vi "QA_Sub.vi"(0 "U":dbl[](array[numeric]) format="%.2f", 2 "W":dbl[](array[numeric]) format="%.2f", 3 "T":dbl[](array[numeric]) format="%.2f") -> ()   [LabVIEW 2010]
uses:
  Controls/Analysis_type_Enum.ctl
  <vilib>/Utility/file.llb/Write To Spreadsheet File (DBL).vi
  <vilib>/Analysis/NI_AALBase.lvlib
panel:
  out "Loop Frame 1":i32
  out "Loop Frame 0":i32
  out "Analysis type":T1
  in  "LDA data?":bool
  in  "QA results file":path
  out "Quadrant shear totals":dbl[](array[numeric]) format="%.3f"
  out "Quadrant 'Hits' Count":dbl[](array[numeric])
  out "u'w' (bar) total":dbl format="%.3f"
  in  "H":dbl format="%.2f"
  out "XY Graph":cluster{dbl[], dbl[]}(graph)
  in  "u', w' data file":path
  # "Quadrant Analysis Subroutine for Two-Component Velocity Data"
  # "Version 1.2 -RR"
  # "Threshold,"
  # "- FOR MANUAL ENTRY -"
  # "- FOR PLUG-IN USE -"
  # "- FILES TO CREATE -"
  # "- ANALYSIS (OUTPUT) -"
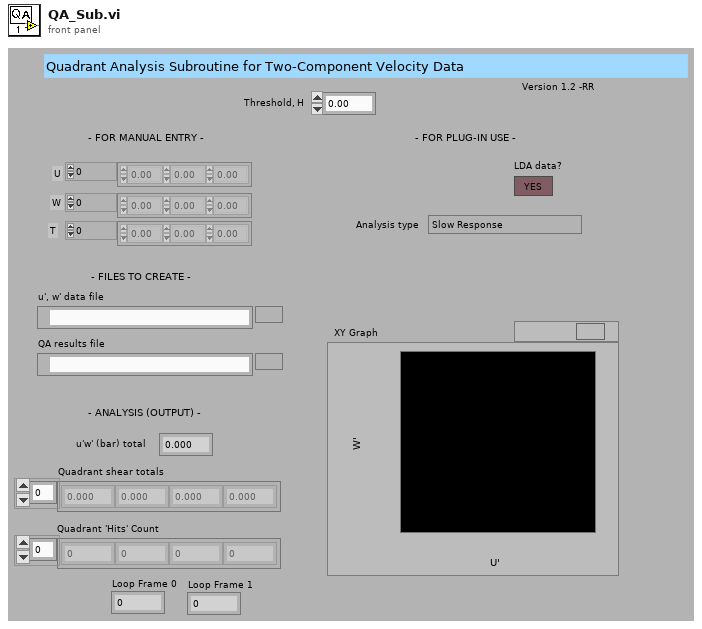
[diagram p1: front panel]
types:
  T1 = typedef "Analysis_type_Enum.ctl" = enum16{"Slow Response", "Fast Response", "Weighted Fast Response", "Fast FID", "Weighted Fast FID", "Cross Wire", "Weighted Cross Wire", "Weighted LDA"}
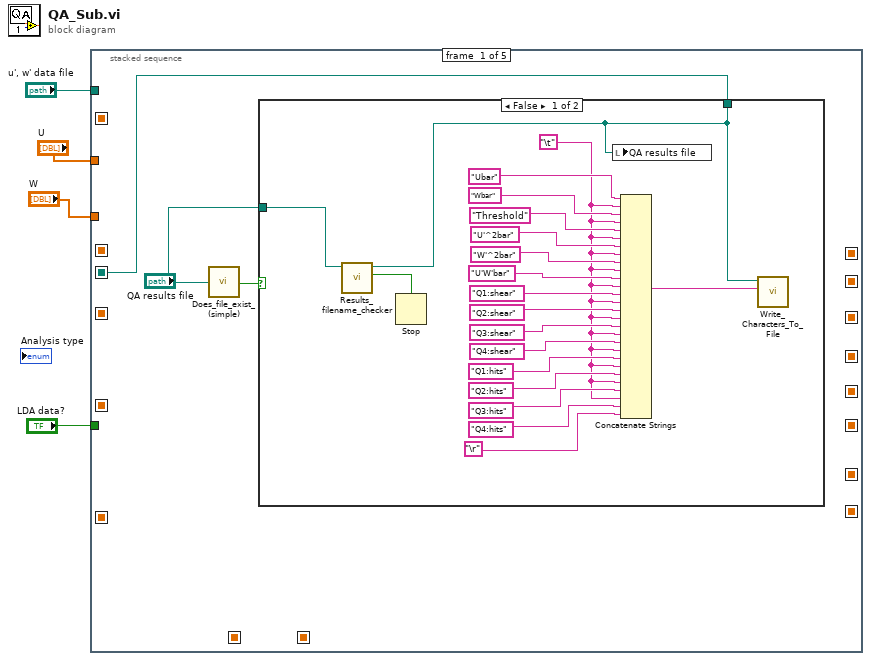
[diagram p0: block diagram]
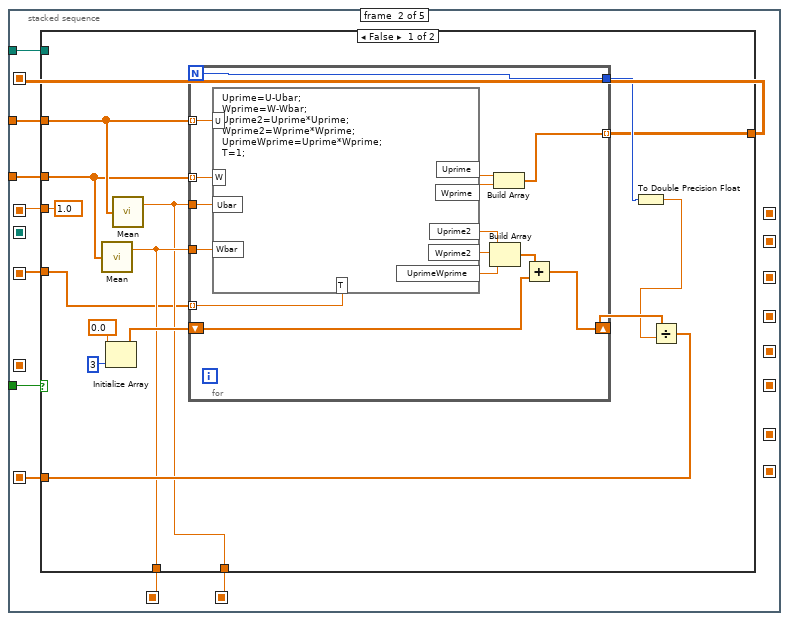
[diagram p3: hidden frame]
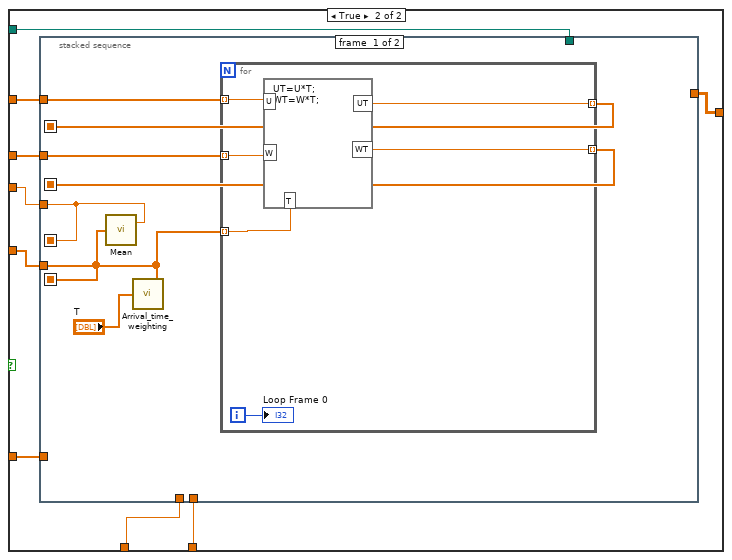
[diagram p4: hidden frame]
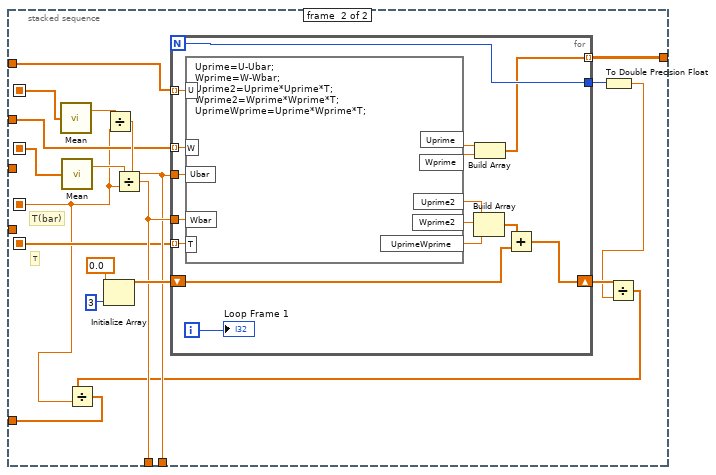
[diagram p5: hidden frame]
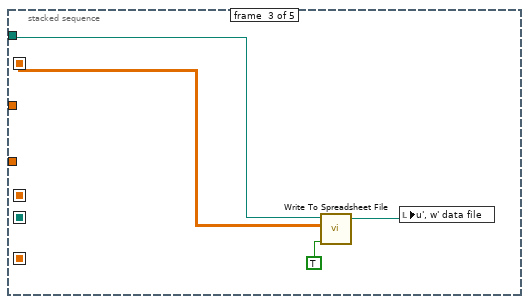
[diagram p6: hidden frame]
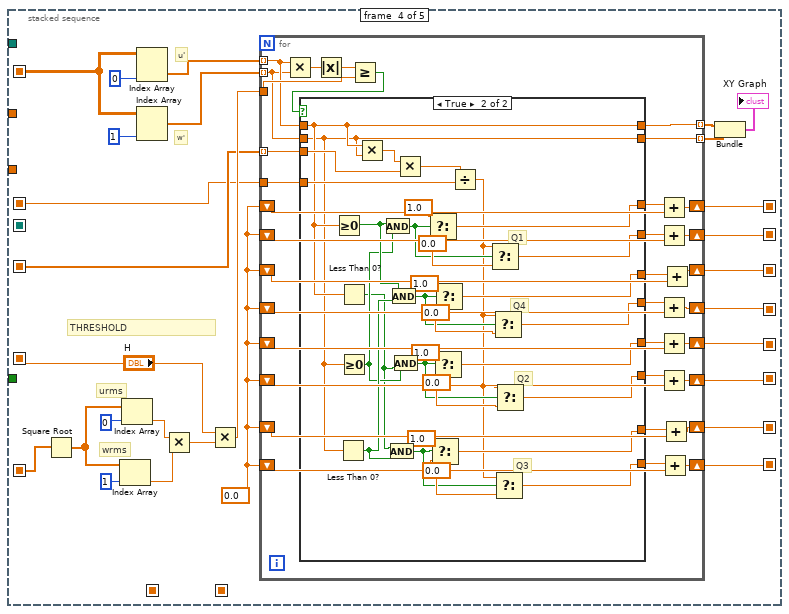
[diagram p7: hidden frame]
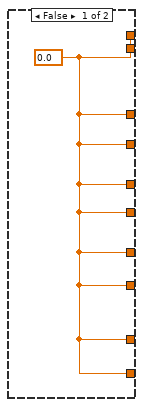
[diagram p8: hidden frame]
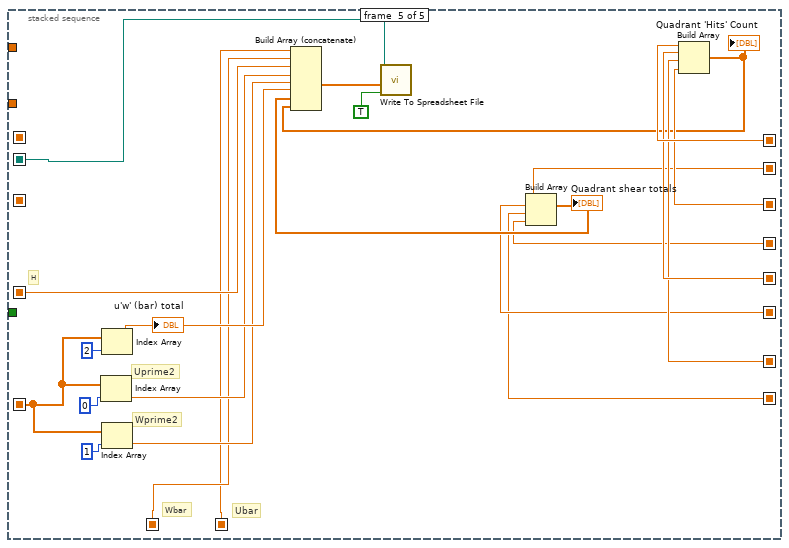
[diagram p9: hidden frame]
diagram:
  n1 = stacked-sequence {
    seq-local: [_ w37 _ _ _] -> [_ _ _ w133 w232]
    seq-local: [_ _ _ w140 _] -> [_ _ _ _ w238]
    seq-local: [_ _ _ w141 _] -> [_ _ _ _ w244]
    seq-local: [_ _ _ w139 _] -> [_ _ _ _ w241]
    seq-local: [_ _ _ w138 _] -> [_ _ _ _ w235]
    seq-local: [_ _ _ w137 _] -> [_ _ _ _ w243]
    seq-local: [_ _ _ w136 _] -> [_ _ _ _ w237]
    seq-local: [_ _ _ w135 _] -> [_ _ _ _ w242]
    seq-local: [_ _ _ w134 _] -> [_ _ _ _ w236]
    seq-local: [_ _ _ "H" _] -> [_ _ _ _ w231]
    seq-local: [_ w35 _ _ _] -> [_ _ _ _ w225]
    seq-local: [_ w34 _ _ _] -> [_ _ _ _ w224]
    seq-local: [_ w33 _ _ _] -> [_ _ _ w130 _]
    seq-local: [_ w32 _ _ _] -> [_ _ _ w131 _]
    seq-local: [_ w31 _ _ _] -> [_ _ w127 w129 _]
    seq-local: [w5 _ _ _ _] -> [_ _ _ _ w223]
    tunnel: "u', w' data file" -> [_ w38 w126 _ _]
    tunnel: "LDA data?" -> [_ w36 _ _ _]
    tunnel: "U" -> [_ w30 _ _ _]
    tunnel: "W" -> [_ w29 _ _ _]
    frame #0 {
      n2 = call "Does_file_exist_(simple).vi"("Pathname"="QA results file") -> ("exists?"=w7:bool)
      n3 = case shown="False" w7 {
        tunnel: [w9 w28] -> w5
        tunnel: "QA results file" -> [w10 w28]
        frame False {
          w12 = "\t"
          n4 = call "Results_filename_checker.vi"("Results file"=w10) -> ("cancelled"=w8:bool, "Results file output"=w9:path)  [unwired: 4 in, 2 out]
          n5 = Stop(stop? (T)=w8) -> ()
          n6 = local write "QA results file"(w9) -> ()
          n7 = Concatenate Strings("Ubar", w12, "Wbar", w12, "Threshold", w12, "U'^2bar", w12, "W'^2bar", w12, "U'W'bar", w12, "Q1:shear", w12, "Q2:shear", w12, "Q3:shear", w12, "Q4:shear", w12, "Q1:hits", w12, "Q2:hits", w12, "Q3:hits", w12, "Q4:hits", "\r") -> (w11:string)
          n8 = call "Write_Characters_To_File.vi"("file path (dialog if empty)"=w9, "character string"=w11) -> ()  [unwired: 6 in, 1 out]
        }
        frame True {
        }
      }
    }
    frame #1 {
      n9 = case shown="False" w36 {
        tunnel: w38 -> [_ w76]
        tunnel: [w48 w71] -> w37
        tunnel: w30 -> [w45 w75]
        tunnel: w29 -> [w44 w74]
        tunnel: [w43 w73] -> w35
        tunnel: [w42 w72] -> w34
        tunnel: [1.0 w70] -> w33
        tunnel: [w40 w69] -> w32
        tunnel: [w39 w68] -> w31
        frame False {
          n10 = call <vilib>:"Mean.vi"("X"=w44) -> ("mean"=w43:dbl)  [unwired: 1 out]
          n11 = Initialize Array(0.0, 3) -> (w51:dbl[])
          n12 = call <vilib>:"Mean.vi"("X"=w45) -> ("mean"=w42:dbl)  [unwired: 1 out]
          n13 = for {
            N -> [w58]
            tunnel: w45 -> [w67] mode=indexing
            tunnel: w44 -> [w66] mode=indexing
            shift-right: [w59] -> w49
            shift-left: w51 -> [w60]
            tunnel: [w58] -> w47
            tunnel: w42 -> [w56]
            tunnel: w43 -> [w55]
            tunnel: [w54] -> w40 mode=indexing
            tunnel: [w53] -> w39 mode=indexing
            n14 = formula code="Uprime=U-Ubar;\nWprime=W-Wbar;\nUprime2=Uprime*Uprime;\nWprime2=Wprime*Wprime;\nUprimeWprime=Uprime*Wprime;\nT=1;"("W"=w66, "U"=w67, "Ubar"=w56, "Wbar"=w55) -> ("Uprime"=w65:dbl, "Wprime"=w64:dbl, "Uprime2"=w63:dbl, "Wprime2"=w62:dbl, "UprimeWprime"=w57:dbl, "T"=w54:dbl)
            n15 = Build Array(w63, w62, w57) -> (w61:dbl[])
            n16 = Build Array(w65, w64) -> (w53:dbl[])
            n17 = Add(x=w61, y=w60) -> (x+y=w59:dbl[])
          }
          n18 = To Double Precision Float(number=w47) -> (double precision float=w46:dbl)
          n19 = Divide(x=w49, y=w46) -> (x/y=w48:dbl[])
        }
        frame True {
          n20 = stacked-sequence {
            seq-local: [w81 _] -> [_ w104]
            seq-local: [w80 _] -> [_ w105]
            seq-local: [w79 _] -> [_ w93]
            seq-local: [w78 _] -> [_ w97]
            tunnel: w76 -> [_ _]
            tunnel: w75 -> [w83 w99]
            tunnel: w74 -> [w82 w98]
            tunnel: [_ w103] -> w73
            tunnel: [_ w100] -> w72
            tunnel: [_ w92] -> w71
            tunnel: [w79 _] -> w70
            tunnel: [w78 _] -> w69
            tunnel: [_ w90] -> w68
            frame #0 {
              n21 = call "Arrival_time_weighting.vi"("Arrival times"="T") -> ("Weighting"=w78:dbl[])
              n22 = call <vilib>:"Mean.vi"("X"=w78) -> ("mean"=w79:dbl)  [unwired: 1 out]
              n23 = for {
                tunnel: w83 -> [w89] mode=indexing
                tunnel: w82 -> [w88] mode=indexing
                tunnel: w78 -> [w87] mode=indexing
                tunnel: [w86] -> w81 mode=indexing
                tunnel: [w85] -> w80 mode=indexing
                i -> [w84]
                n24 = formula code="UT=U*T;\nWT=W*T;"("T"=w87, "U"=w89, "W"=w88) -> ("UT"=w86:dbl, "WT"=w85:dbl)
                "Loop Frame 0" <- w84
              }
            }
            frame #1 {
              # "T"
              # "T(bar)"
              n25 = call <vilib>:"Mean.vi"("X"=w104) -> ("mean"=w102:dbl)  [unwired: 1 out]
              n26 = call <vilib>:"Mean.vi"("X"=w105) -> ("mean"=w101:dbl)  [unwired: 1 out]
              n27 = Initialize Array(0.0, 3) -> (w106:dbl[])
              n28 = Divide(x=w102, y=w93) -> (x/y=w100:dbl)
              n29 = Divide(x=w101, y=w93) -> (x/y=w103:dbl)
              n30 = for {
                N -> [w115]
                tunnel: w99 -> [w124] mode=indexing
                tunnel: w98 -> [w123] mode=indexing
                shift-right: [w116] -> w95
                shift-left: w106 -> [w117]
                tunnel: [w115] -> w96
                tunnel: w100 -> [w113]
                tunnel: w103 -> [w112]
                tunnel: w97 -> [w111] mode=indexing
                tunnel: [w110] -> w90 mode=indexing
                i -> [w109]
                n31 = formula code="Uprime=U-Ubar;\nWprime=W-Wbar;\nUprime2=Uprime*Uprime*T;\nWprime2=Wprime*Wprime*T;\nUprimeWprime=Uprime*Wprime*T;"("W"=w123, "U"=w124, "Ubar"=w113, "Wbar"=w112, "T"=w111) -> ("Uprime"=w122:dbl, "Wprime"=w121:dbl, "Uprime2"=w120:dbl, "Wprime2"=w119:dbl, "UprimeWprime"=w114:dbl)
                n32 = Build Array(w120, w119, w114) -> (w118:dbl[])
                n33 = Build Array(w122, w121) -> (w110:dbl[])
                n34 = Add(x=w118, y=w117) -> (x+y=w116:dbl[])
                "Loop Frame 1" <- w109
              }
              n35 = To Double Precision Float(number=w96) -> (double precision float=w94:dbl)
              n36 = Divide(x=w95, y=w94) -> (x/y=w91:dbl[])
              n37 = Divide(x=w91, y=w93) -> (x/y=w92:dbl[])
            }
          }
        }
      }
    }
    frame #2 {
      n38 = call-poly <vilib>:"Write To Spreadsheet File.vi"("append to file? (new file:F)"=TRUE, "2D data"=w127, "file path (dialog if empty)"=w126) -> ("new file path (Not A Path if cancelled)"=w125:path)  [unwired: 5 in]
      n39 = local write "u', w' data file"(w125) -> ()
    }
    frame #3 {
      w132 = 0.0
      # "THRESHOLD"
      # "wrms"
      # "urms"
      # "w'"
      # "u'"
      n40 = Square Root(x=w133) -> (sqrt(x)=w154:dbl[])
      n41 = Index Array(array=w154, index=1) -> (element=w150:dbl)
      n42 = Index Array(array=w154, index=0) -> (element=w151:dbl)
      n43 = Index Array(array=w129, index (col)=0) -> (element=w147:dbl[])  [unwired: 1 in]
      n44 = Index Array(array=w129, index (col)=1) -> (element=w146:dbl[])  [unwired: 1 in]
      n45 = Multiply(x=w151, y=w150) -> (x*y=w148:dbl)
      n46 = Multiply(x="H", y=w148) -> (x*y=w145:dbl)
      n47 = for {
        tunnel: w147 -> [w186] mode=indexing
        tunnel: w146 -> [w185] mode=indexing
        tunnel: w145 -> [w188]
        tunnel: [w184] -> w144 mode=indexing
        tunnel: [w183] -> w143 mode=indexing
        shift-right: [w175] -> w140
        shift-left: w132 -> [w165]
        shift-right: [w182] -> w138
        shift-left: w132 -> [w163]
        shift-right: [w181] -> w136
        shift-left: w132 -> [w161]
        shift-right: [w180] -> w134
        shift-left: w132 -> [w159]
        shift-right: [w167] -> w141
        shift-left: w132 -> [w166]
        shift-right: [w174] -> w139
        shift-left: w132 -> [w164]
        shift-right: [w173] -> w137
        shift-left: w132 -> [w162]
        shift-right: [w168] -> w135
        shift-left: w132 -> [w160]
        tunnel: w131 -> [w158] mode=indexing
        tunnel: w130 -> [w157]
        n48 = Multiply(x=w186, y=w185) -> (x*y=w190:dbl)
        n49 = Absolute Value(x=w190) -> (abs(x)=w189:dbl)
        n50 = Greater Or Equal?(x=w189, y=w188) -> (x >= y?=w187:bool)
        n51 = case shown="True" w187 {
          tunnel: w186 -> [_ w195]
          tunnel: w185 -> [_ w194]
          tunnel: [w191 w195] -> w184
          tunnel: [w191 w194] -> w183
          tunnel: [w191 w206] -> w179
          tunnel: [w191 w205] -> w178
          tunnel: [w191 w204] -> w177
          tunnel: [w191 w203] -> w176
          tunnel: [w191 w202] -> w172
          tunnel: [w191 w201] -> w171
          tunnel: [w191 w200] -> w170
          tunnel: [w191 w199] -> w169
          tunnel: w158 -> [_ w196]
          tunnel: w157 -> [_ w198]
          frame False {
            w191 = 0.0
          }
          frame True {
            w219 = 0.0
            w220 = 0.0
            w221 = 0.0
            w222 = 0.0
            # "Q3"
            # "Q2"
            # "Q4"
            # "Q1"
            n52 = Greater Or Equal To 0?(x=w195) -> (x >= 0?=w214:bool)
            n53 = Less Than 0?(x=w194) -> (x < 0?=w213:bool)
            n54 = Less Than 0?(x=w195) -> (x < 0?=w211:bool)
            n55 = Greater Or Equal To 0?(x=w194) -> (x >= 0?=w212:bool)
            n56 = Multiply(x=w195, y=w194) -> (x*y=w193:dbl)
            n57 = And(x=w214, y=w212) -> (x .and. y?=w210:bool)
            n58 = And(x=w211, y=w213) -> (x .and. y?=w207:bool)
            n59 = And(x=w214, y=w213) -> (x .and. y?=w209:bool)
            n60 = And(x=w212, y=w211) -> (x .and. y?=w208:bool)
            n61 = Multiply(x=w193, y=w196) -> (x*y=w192:dbl)
            n62 = Select(t=1.0, s=w210, f=w222) -> (s? t:f=w202:dbl)
            n63 = Select(t=1.0, s=w207, f=w219) -> (s? t:f=w199:dbl)
            n64 = Select(t=1.0, s=w208, f=w220) -> (s? t:f=w200:dbl)
            n65 = Select(t=1.0, s=w209, f=w221) -> (s? t:f=w201:dbl)
            n66 = Divide(x=w192, y=w198) -> (x/y=w197:dbl)
            n67 = Select(t=w197, s=w210, f=w222) -> (s? t:f=w206:dbl)
            n68 = Select(t=w197, s=w209, f=w221) -> (s? t:f=w205:dbl)
            n69 = Select(t=w197, s=w207, f=w219) -> (s? t:f=w203:dbl)
            n70 = Select(t=w197, s=w208, f=w220) -> (s? t:f=w204:dbl)
          }
        }
        n71 = Add(x=w172, y=w166) -> (x+y=w167:dbl)
        n72 = Add(x=w179, y=w165) -> (x+y=w175:dbl)
        n73 = Add(x=w178, y=w163) -> (x+y=w182:dbl)
        n74 = Add(x=w170, y=w162) -> (x+y=w173:dbl)
        n75 = Add(x=w177, y=w161) -> (x+y=w181:dbl)
        n76 = Add(x=w176, y=w159) -> (x+y=w180:dbl)
        n77 = Add(x=w169, y=w160) -> (x+y=w168:dbl)
        n78 = Add(x=w171, y=w164) -> (x+y=w174:dbl)
      }
      n79 = Bundle(w144, w143) -> (→"XY Graph":cluster{dbl[], dbl[]})  [unwired: 1 in]
    }
    frame #4 {
      # "Wprime2"
      # "Uprime2"
      # "H"
      # "Wbar"
      # "Ubar"
      n80 = Index Array(array=w232, index=0) -> (element=w230:dbl)
      n81 = Index Array(array=w232, index=2) -> (element=w239:dbl)
      "u'w' (bar) total" <- w239
      n82 = Index Array(array=w232, index=1) -> (element=w229:dbl)
      n83 = Build Array(w238, w237, w236, w235) -> (w240:dbl[])
      "Quadrant shear totals" <- w240
      n84 = Build Array(w244, w243, w242, w241) -> (w228:dbl[])
      "Quadrant 'Hits' Count" <- w228
      n85 = Build Array (concatenate)(w224, w225, w231, w230, w229, w239, w240, w228) -> (w226:dbl[])
      n86 = call-poly <vilib>:"Write To Spreadsheet File.vi"("append to file? (new file:F)"=TRUE, "1D data"=w226, "file path (dialog if empty)"=w223) -> ()  [unwired: 5 in, 1 out]
    }
  }
